vi "FlushAndShutOff_v01.vi"(2 "Debug Mode":bool, 3 "Elapsed Time(s)":dbl, 4 "State":enum16{"Edit", "Start", "Run", "End", "Idle"}(ring), 5 "Argument List In":string[](array[string])) -> (0 "Status Out":string, 1 "Argument List Out":string[](array[string]))   [LabVIEW 2011]
panel:
  out "first":bool=TRUE
  out "total time":dbl
  out "is OK?":bool
  out "AsH3?":bool
  out "PH3?":bool
  out "In?":bool
  out "Ga?":bool
  out "Al?":bool
  in  "AsH3 Flow":dbl caption="AsH3 Flow (0-10 sccm)" format="%.2f"
  in  "P Flow":dbl caption="P Flow (0-100 sccm)" format="%.2f"
  in  "In Flow":dbl caption="In Flow (0-100 sscm)" format="%.2f"
  in  "Ga Flow":dbl caption="Ga Flow (0-10 sscm)" format="%.2f"
  in  "Al Flow":dbl caption="Al Flow (0-100 sscm)" format="%.2f"
  in  "Cancel":bool
  in  "OK":bool
  out "tTotal(s) 2":dbl
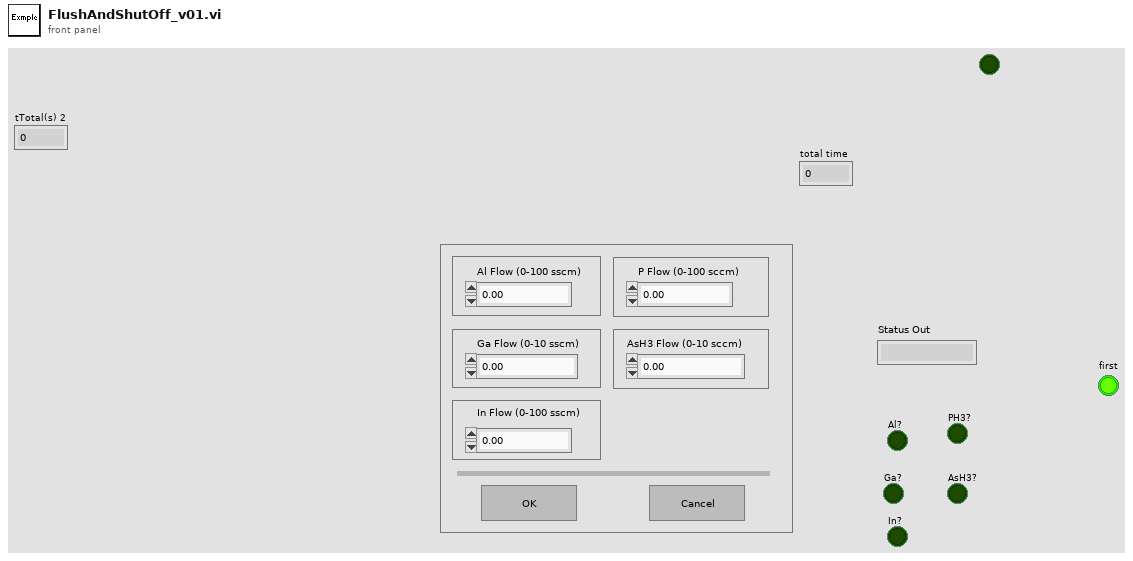
[diagram p1: front panel]
types:
  T1 = enum16{"Discrete", "Continuous", "Instantaneous", "Finite"}
  T2 = enum32{"Invalid", "Default", "Floating", "Floating/Auto-Hide", "Modal"}
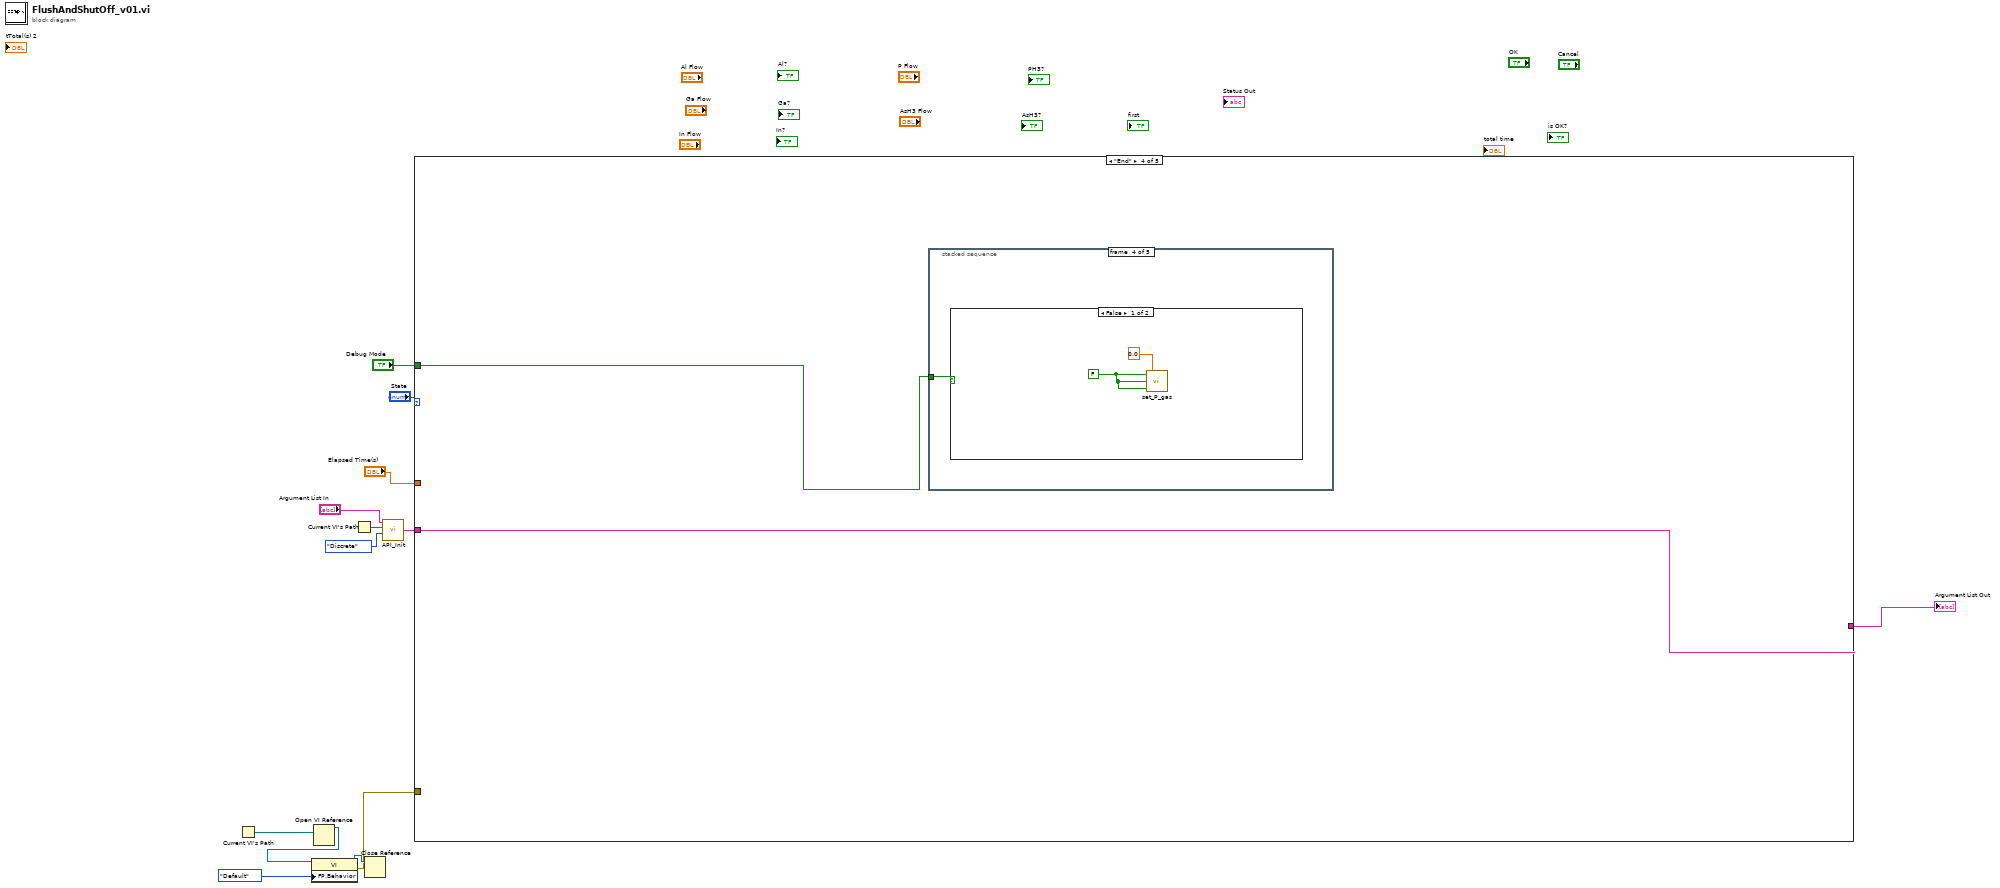
[diagram p0: block diagram]
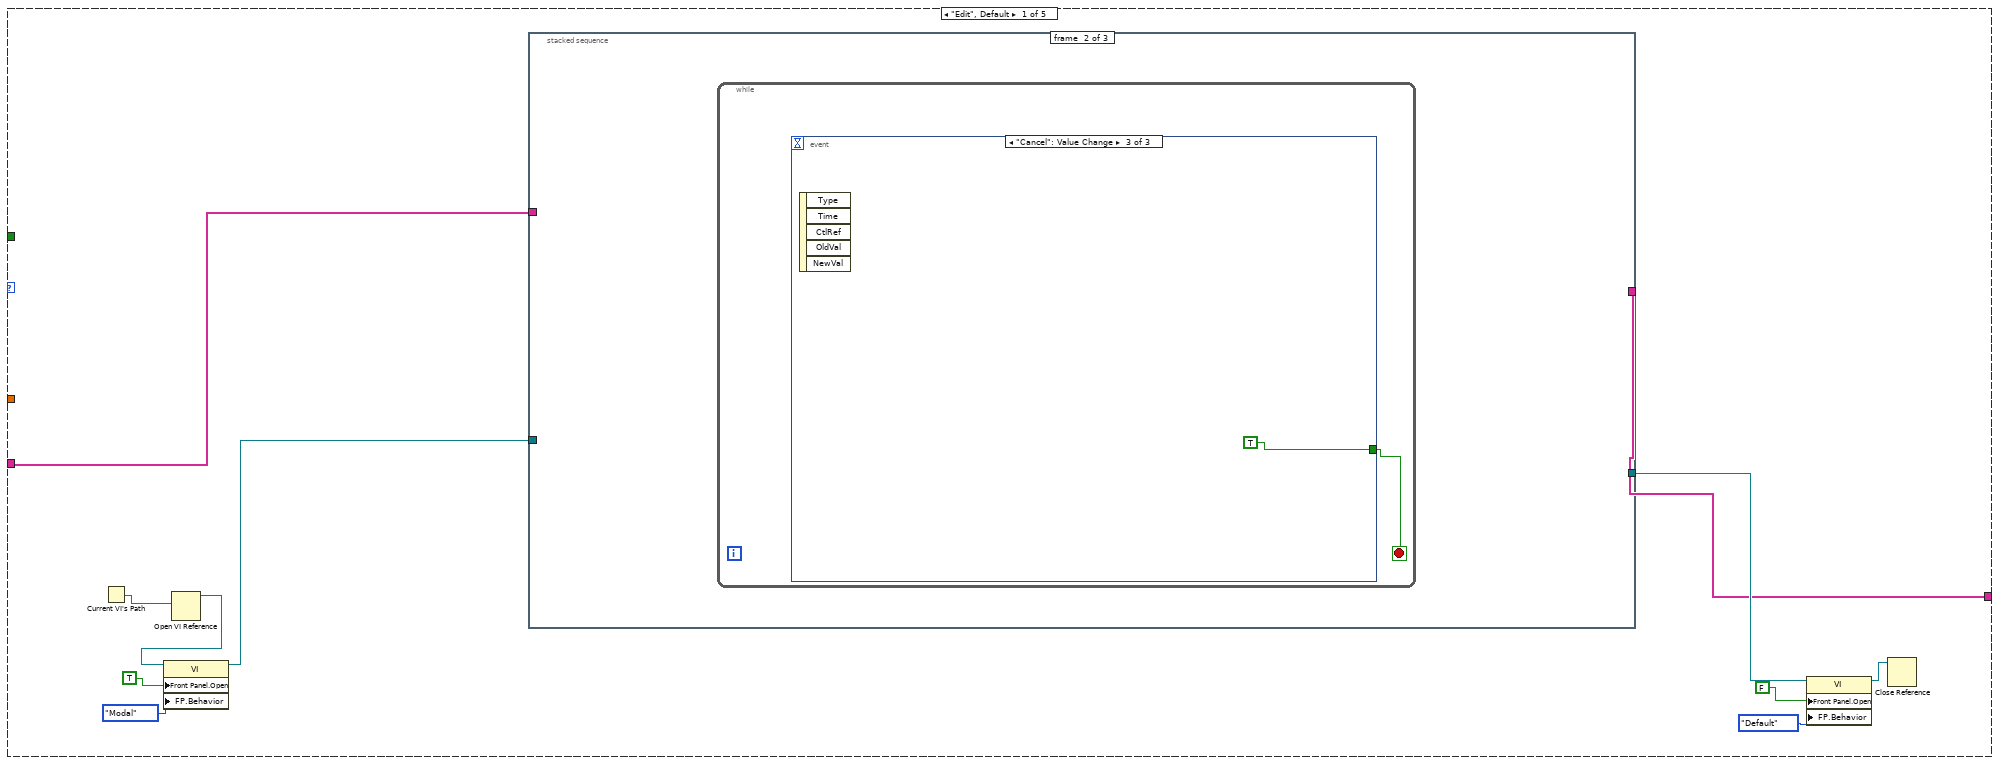
[diagram p2: hidden frame]
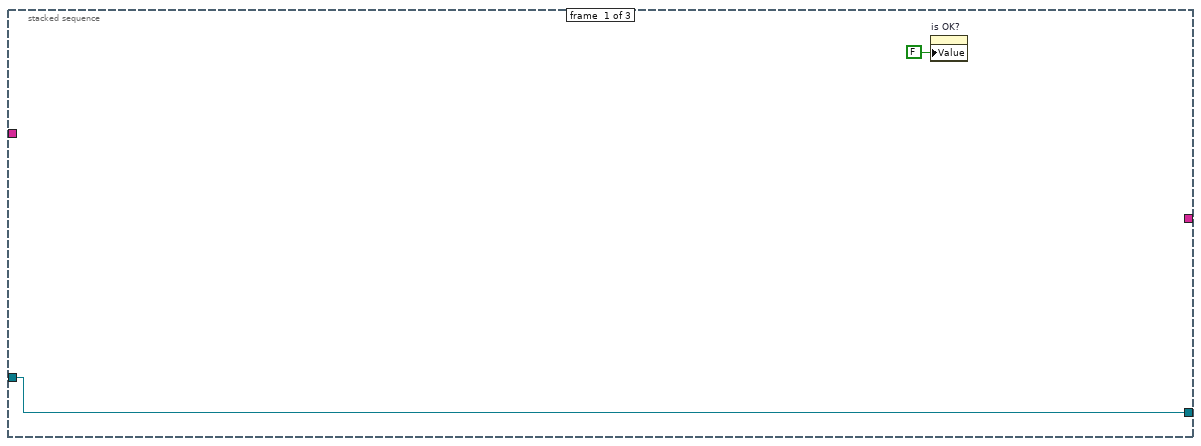
[diagram p3: hidden frame]
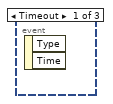
[diagram p4: hidden frame]
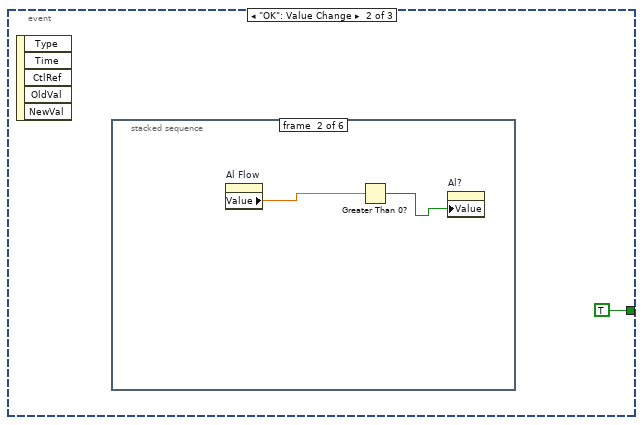
[diagram p5: hidden frame]
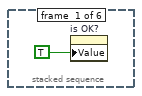
[diagram p6: hidden frame]
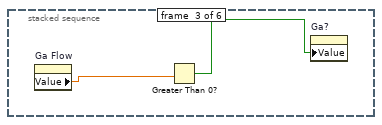
[diagram p7: hidden frame]
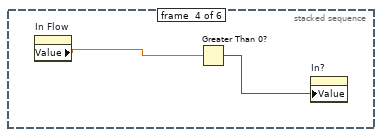
[diagram p8: hidden frame]
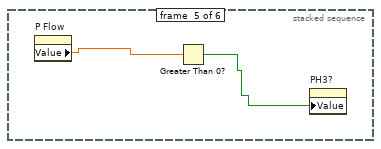
[diagram p9: hidden frame]
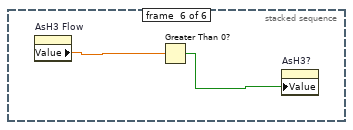
[diagram p10: hidden frame]
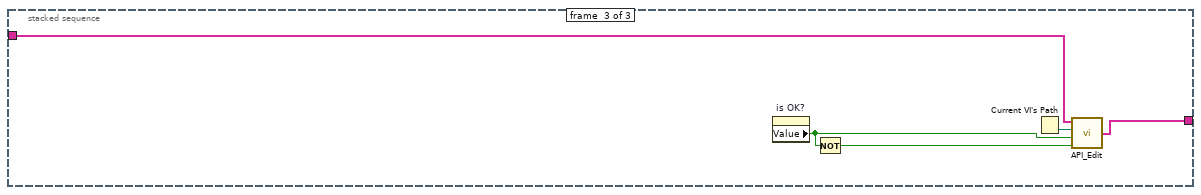
[diagram p11: hidden frame]
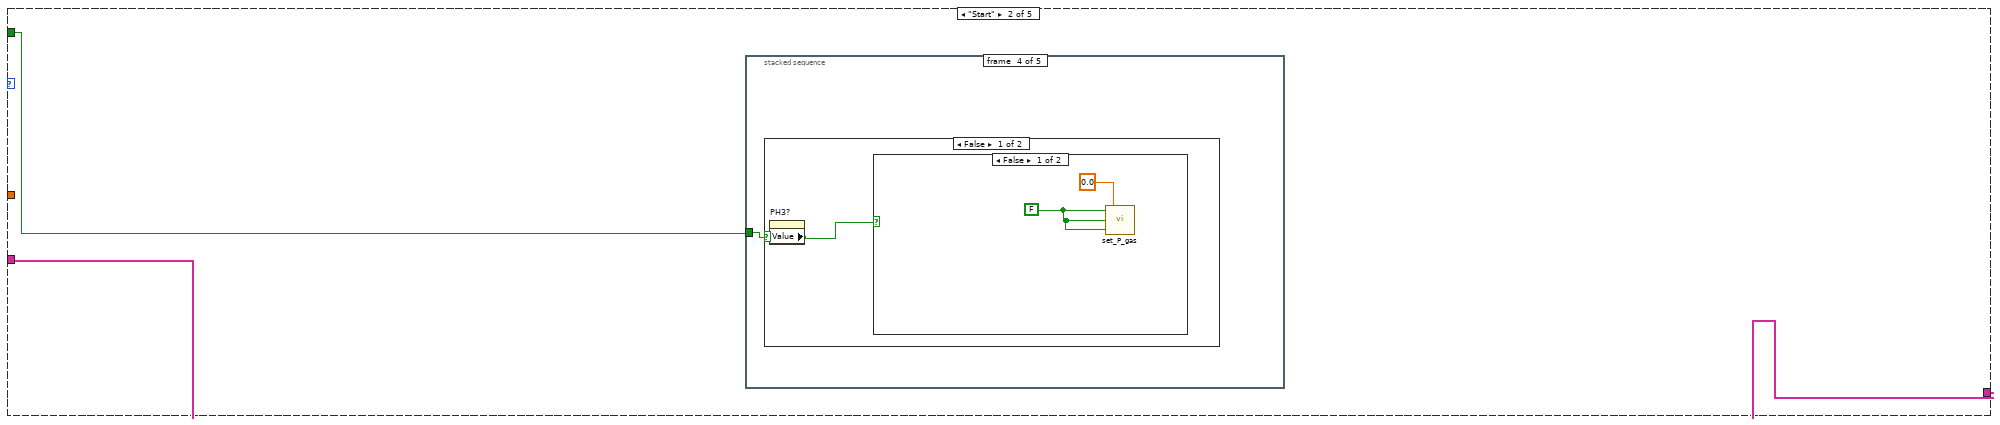
[diagram p12: hidden frame]
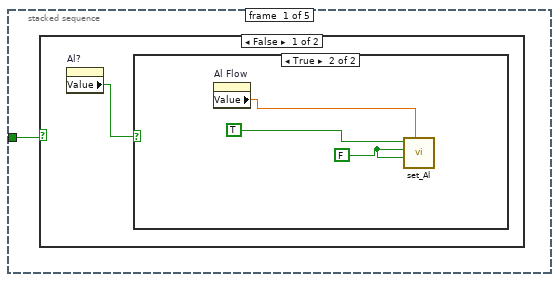
[diagram p13: hidden frame]
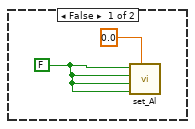
[diagram p14: hidden frame]
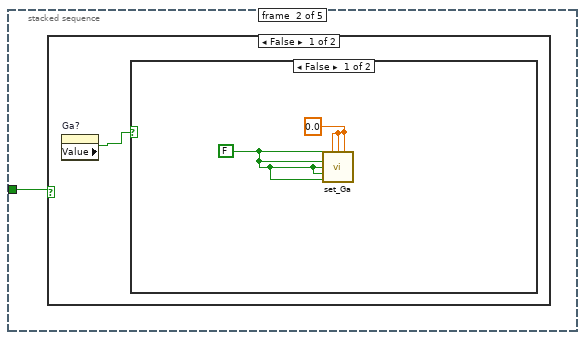
[diagram p16: hidden frame]
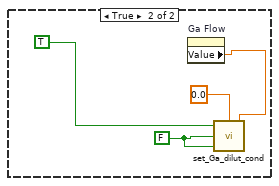
[diagram p17: hidden frame]
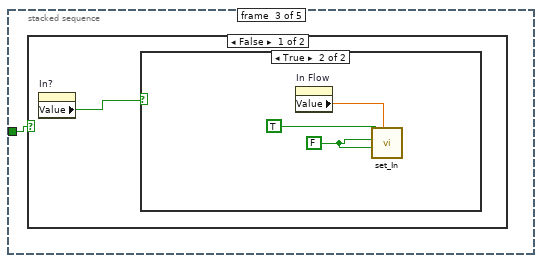
[diagram p19: hidden frame]
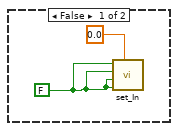
[diagram p20: hidden frame]
diagram:
  n1 = Current VI's Path() -> (path=w9:path)
  n2 = Open VI Reference(vi path=w9) -> (vi reference=w8:refnum<vi>)  [unwired: 1 in, 5 out]
  n3 = property class="VI"(reference=w8, "FP.Behavior"=T2."Default" ("Front Panel Window:Behavior")) -> (reference out=w6:refnum<vi>, error out=w5:errorcluster)  [unwired: 1 in]
  n4 = Current VI's Path() -> (path=w4:path)
  n5 = Close Reference(reference=w6) -> ()  [unwired: 1 in, 1 out]
  n6 = call "API_Init.vi"("API Mode"=T1."Discrete", "VI Path"=w4, "Argument List In"="Argument List In") -> ("Argument List Out"=w1:string[])  [unwired: 1 in]
  n7 = case shown="\"End\"" "State" {
    tunnel: "Debug Mode" -> [_ w47 _ w85 _]
    tunnel: "Elapsed Time(s)" -> [_ _ _ _ _]
    tunnel: w1 -> [w15 w46 w84 w86 w102]
    tunnel: [w14 w46 w84 w86 w102] -> w10
    tunnel: w5 -> [_ _ _ _ _]
    frame "Edit", Default {
      n8 = Current VI's Path() -> (path=w20:path)
      n9 = Open VI Reference(vi path=w20) -> (vi reference=w19:refnum<vi>)  [unwired: 1 in, 5 out]
      n10 = property class="VI"(reference=w19, "Front Panel.Open"=TRUE ("Front Panel Window:Open"), "FP.Behavior"=T2."Modal" ("Front Panel Window:Behavior")) -> (reference out=w18:refnum<vi>)  [unwired: 1 in, 1 out]
      n11 = stacked-sequence {
        tunnel: w15 -> [_ _ w41]
        tunnel: w18 -> [w26 _ _]
        tunnel: [w26 _ _] -> w22
        tunnel: [_ _ w43] -> w14
        frame #0 {
          n12 = property on="is OK?" class="Bool (strict)"("Value"=FALSE ("is OK?")) -> ()  [unwired: 2 in, 2 out]
        }
        frame #1 {
          n13 = while {
            stop <- w27 stop-if-true
            n14 = event shown="[2] \"Cancel\": Value Change" {
              selector: _ -> [_ _ _]
              dyn-events: _ -> [_ _ _]
              timeout: _ -> [_ _ _]
              tunnel: [_ TRUE TRUE] -> w27
              event Timeout {
                n15 = event-data() -> ()  [unwired: 1 in, 2 out]
              }
              event "OK": Value Change {
                n16 = event-data() -> ()  [unwired: 1 in, 5 out]
                n17 = stacked-sequence {
                  frame #0 {
                    n18 = property on="is OK?" class="Bool (strict)"("Value"=TRUE ("is OK?")) -> ()  [unwired: 2 in, 2 out]
                  }
                  frame #1 {
                    n19 = property on="Al Flow" class="DigNum (strict)"() -> ("Value"=w31:dbl)  [unwired: 2 in, 2 out]
                    n20 = Greater Than 0?(x=w31) -> (x > 0?=w30:bool)
                    n21 = property on="Al?" class="Bool (strict)"("Value"=w30) -> ()  [unwired: 2 in, 2 out]
                  }
                  frame #2 {
                    n22 = property on="Ga Flow" class="DigNum (strict)"() -> ("Value"=w33:dbl)  [unwired: 2 in, 2 out]
                    n23 = Greater Than 0?(x=w33) -> (x > 0?=w32:bool)
                    n24 = property on="Ga?" class="Bool (strict)"("Value"=w32) -> ()  [unwired: 2 in, 2 out]
                  }
                  frame #3 {
                    n25 = property on="In Flow" class="DigNum (strict)"() -> ("Value"=w35:dbl)  [unwired: 2 in, 2 out]
                    n26 = Greater Than 0?(x=w35) -> (x > 0?=w34:bool)
                    n27 = property on="In?" class="Bool (strict)"("Value"=w34) -> ()  [unwired: 2 in, 2 out]
                  }
                  frame #4 {
                    n28 = property on="P Flow" class="DigNum (strict)"() -> ("Value"=w37:dbl)  [unwired: 2 in, 2 out]
                    n29 = Greater Than 0?(x=w37) -> (x > 0?=w36:bool)
                    n30 = property on="PH3?" class="Bool (strict)"("Value"=w36) -> ()  [unwired: 2 in, 2 out]
                  }
                  frame #5 {
                    n31 = property on="AsH3 Flow" class="DigNum (strict)"() -> ("Value"=w39:dbl)  [unwired: 2 in, 2 out]
                    n32 = Greater Than 0?(x=w39) -> (x > 0?=w38:bool)
                    n33 = property on="AsH3?" class="Bool (strict)"("Value"=w38) -> ()  [unwired: 2 in, 2 out]
                  }
                }
              }
              event "Cancel": Value Change {
                n34 = event-data() -> ()  [unwired: 1 in, 5 out]
              }
            }
          }
        }
        frame #2 {
          n35 = property on="is OK?" class="Bool (strict)"() -> ("Value"=w42:bool)  [unwired: 2 in, 2 out]
          n36 = Not(x=w42) -> (.not. x?=w45:bool)
          n37 = Current VI's Path() -> (path=w44:path)
          n38 = call "API_Edit.vi"("Cancel"=w45, "OK"=w42, "VI Path"=w44, "Argument List In"=w41) -> ("Argument List Out"=w43:string[])
        }
      }
      n39 = property class="VI"(reference=w22, "Front Panel.Open"=FALSE ("Front Panel Window:Open"), "FP.Behavior"=T2."Default" ("Front Panel Window:Behavior")) -> (reference out=w23:refnum<vi>)  [unwired: 1 in, 1 out]
      n40 = Close Reference(reference=w23) -> ()  [unwired: 1 in, 1 out]
    }
    frame "Start" {
      n41 = stacked-sequence {
        tunnel: w47 -> [w48 w55 w63 w70 w77]
        frame #0 {
          n42 = case shown="False" w48 {
            frame False {
              n43 = property on="Al?" class="Bool (strict)"() -> ("Value"=w49:bool)  [unwired: 2 in, 2 out]
              n44 = case shown="True" w49 {
                frame False {
                  w50 = FALSE ("Al Active")
                  n45 = call "set_Al.vi"("ALMFC1"=0.0 ("Aluminum Flow"), "Remote"=w50, "Run"=w50, "Bubbler In"=w50, "Active"=w50) -> ()  [unwired: 5 out]
                }
                frame True {
                  w52 = FALSE ("Al Bubbler")
                  n46 = property on="Al Flow" class="DigNum (strict)"() -> ("Value"=w53:dbl)  [unwired: 2 in, 2 out]
                  n47 = call "set_Al.vi"("ALMFC1"=w53, "Run"=w52, "Bubbler In"=w52, "Active"=TRUE ("Al Active")) -> ()  [unwired: 1 in, 5 out]
                }
              }
            }
            frame True {
            }
          }
        }
        frame #1 {
          n48 = case shown="False" w55 {
            frame False {
              n49 = property on="Ga?" class="Bool (strict)"() -> ("Value"=w56:bool)  [unwired: 2 in, 2 out]
              n50 = case shown="False" w56 {
                frame False {
                  w58 = FALSE ("Ga Active")
                  w57 = 0.0 ("Ga Flow 1")
                  n51 = call "set_Ga.vi"("Active"=w58, "GAMFC3"=w57, "GAMFC2"=w57, "GAMFC1"=w57, "Bubbler In"=w58, "H2 Dilute"=w58, "Run"=w58, "Remote"=w58) -> ()  [unwired: 8 out]
                }
                frame True {
                  w59 = FALSE ("Bubbler In")
                  n52 = property on="Ga Flow" class="DigNum (strict)"() -> ("Value"=w60:dbl)  [unwired: 2 in, 2 out]
                  n53 = call "set_Ga_dilut_cond.vi"("Ga flow (0-10 sccm)"=w60, "fDilution"=0.0, "Run"=w59, "Bubbler In"=w59, "Active"=TRUE ("Ga Active")) -> ()
                }
              }
            }
            frame True {
            }
          }
        }
        frame #2 {
          n54 = case shown="False" w63 {
            frame False {
              n55 = property on="In?" class="Bool (strict)"() -> ("Value"=w64:bool)  [unwired: 2 in, 2 out]
              n56 = case shown="True" w64 {
                frame False {
                  w66 = FALSE ("In Remote")
                  n57 = call "set_In.vi"("INMFC1"=0.0 ("Indium Flow"), "Remote"=w66, "Run"=w66, "Bubbler In"=w66, "Active"=w66) -> ()  [unwired: 5 out]
                }
                frame True {
                  w67 = FALSE ("In Bubbler")
                  n58 = property on="In Flow" class="DigNum (strict)"() -> ("Value"=w68:dbl)  [unwired: 2 in, 2 out]
                  n59 = call "set_In.vi"("INMFC1"=w68, "Run"=w67, "Bubbler In"=w67, "Active"=TRUE ("In Run")) -> ()  [unwired: 1 in, 5 out]
                }
              }
            }
            frame True {
            }
          }
        }
        frame #3 {
          n60 = case shown="False" w70 {
            frame False {
              n61 = property on="PH3?" class="Bool (strict)"() -> ("Value"=w71:bool)  [unwired: 2 in, 2 out]
              n62 = case shown="False" w71 {
                frame False {
                  w72 = FALSE ("P_Gas Active")
                  n63 = call "set_P_gas.vi"("Run"=w72, "Gas In"=w72, "Active"=w72, "P_Gas Remote"=w72, "H2 Flush"=w72, "P_Gas Flow"=0.0) -> ()
                }
                frame True {
                  w74 = FALSE ("P_Gas In")
                  w75 = TRUE ("P_Gas Active")
                  n64 = property on="P Flow" class="DigNum (strict)"() -> ("Value"=w76:dbl)  [unwired: 2 in, 2 out]
                  n65 = call "set_P_gas.vi"("Gas In"=w74, "Active"=w75, "P_Gas Remote"=w74, "H2 Flush"=w75, "P_Gas Flow"=w76) -> ()  [unwired: 1 in]
                }
              }
            }
            frame True {
            }
          }
        }
        frame #4 {
          n66 = case shown="False" w77 {
            frame False {
              n67 = property on="AsH3?" class="Bool (strict)"() -> ("Value"=w78:bool)  [unwired: 2 in, 2 out]
              n68 = case shown="True" w78 {
                frame False {
                  w79 = FALSE ("As_Gas Active")
                  n69 = call "set_As_gas.vi"("Active"=w79, "As_Gas Flow"=0.0, "Gas In"=w79, "H2 Flush"=w79, "Run"=w79, "Remote"=w79) -> ()  [unwired: 10 in]
                }
                frame True {
                  w81 = FALSE ("As_Gas In")
                  w82 = TRUE ("As_Gas Active")
                  n70 = property on="AsH3 Flow" class="DigNum (strict)"() -> ("Value"=w83:dbl)  [unwired: 2 in, 2 out]
                  n71 = call "set_As_gas.vi"("Active"=w82, "As_Gas Flow"=w83, "Gas In"=w81, "H2 Flush"=w82, "Run"=w81) -> ()  [unwired: 11 in]
                }
              }
            }
            frame True {
            }
          }
        }
      }
    }
    frame "Run" {
    }
    frame "End" {
      n72 = stacked-sequence {
        tunnel: w85 -> [w87 w90 w93 w96 w99]
        frame #0 {
          n73 = case shown="False" w87 {
            frame False {
              w89 = FALSE ("Al Active")
              n74 = call "set_Al.vi"("ALMFC1"=0.0 ("Aluminum Flow"), "Remote"=w89, "Run"=w89, "Bubbler In"=w89, "Active"=w89) -> ()  [unwired: 5 out]
            }
            frame True {
            }
          }
        }
        frame #1 {
          n75 = case shown="False" w90 {
            frame False {
              w92 = FALSE ("Ga Active")
              w91 = 0.0 ("Ga Flow 1")
              n76 = call "set_Ga.vi"("Active"=w92, "GAMFC3"=w91, "GAMFC2"=w91, "GAMFC1"=w91, "Bubbler In"=w92, "H2 Dilute"=w92, "Run"=w92, "Remote"=w92) -> ()  [unwired: 8 out]
            }
            frame True {
            }
          }
        }
        frame #2 {
          n77 = case shown="False" w93 {
            frame False {
              w95 = FALSE ("In Remote")
              n78 = call "set_In.vi"("INMFC1"=0.0 ("Indium Flow"), "Remote"=w95, "Run"=w95, "Bubbler In"=w95, "Active"=w95) -> ()  [unwired: 5 out]
            }
            frame True {
            }
          }
        }
        frame #3 {
          n79 = case shown="False" w96 {
            frame False {
              w97 = FALSE ("P_Gas Active")
              n80 = call "set_P_gas.vi"("Run"=w97, "Gas In"=w97, "Active"=w97, "P_Gas Remote"=w97, "H2 Flush"=w97, "P_Gas Flow"=0.0) -> ()
            }
            frame True {
            }
          }
        }
        frame #4 {
          n81 = case shown="False" w99 {
            frame False {
              w100 = FALSE ("As_Gas Active")
              n82 = call "set_As_gas.vi"("Active"=w100, "As_Gas Flow"=0.0, "Gas In"=w100, "H2 Flush"=w100, "Run"=w100, "Remote"=w100) -> ()  [unwired: 10 in]
            }
            frame True {
            }
          }
        }
      }
    }
    frame "Idle" {
    }
  }
  "Argument List Out" <- w10
